vi "Accelerometer Gyroscope and Magnetometer.vi"() -> ()   [LabVIEW 2012, in "Phidget Common.lvlib"]
uses:
  <instrlib>/Phidgets/Phidget Common/Phidget Common.lvlib
  <instrlib>/Phidgets/Phidget Magnetometer/Public/MagnetometerClose.vi
  <instrlib>/Phidgets/Phidget Gyroscope/Public/GyroscopeClose.vi
  <instrlib>/Phidgets/Phidget Accelerometer/Public/AccelerometerClose.vi
  <instrlib>/Phidgets/Phidget Gyroscope/Public/GyroscopeStart.vi
  <instrlib>/Phidgets/Phidget Accelerometer/Public/AccelerometerStart.vi
  <instrlib>/Phidgets/Phidget Magnetometer/Public/MagnetometerStart.vi
  <instrlib>/Phidgets/Phidget Accelerometer/Phidget Accelerometer.lvlib
  <instrlib>/Phidgets/Phidget Gyroscope/Phidget Gyroscope.lvlib
  <instrlib>/Phidgets/Phidget Magnetometer/Phidget Magnetometer.lvlib
panel:
  in  "Device Info":T1={"Serial Number"=-1, "Channel"=0, "Port"=0}
  out "FieldStrength":dbl[](array[numeric])
  out "AngularRate":dbl[](array[numeric])
  out "Acceleration":dbl[](array[numeric])
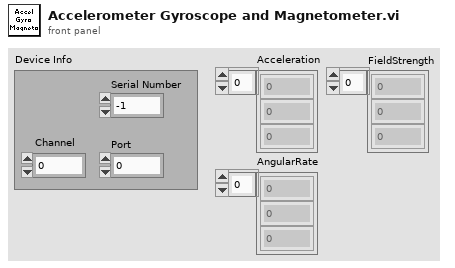
[diagram p1: front panel]
types:
  T1 = cluster{"Serial Number":i32, "Channel":i32, "Port":i32}
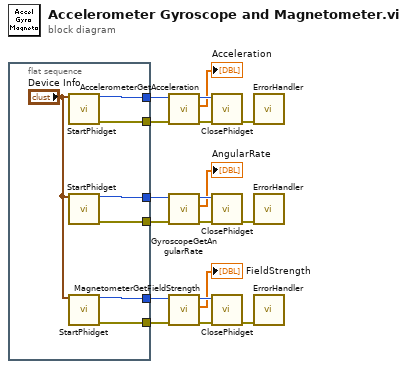
[diagram p0: block diagram]
diagram:
  n1 = flat-sequence {
    tunnel: [w19] -> w18
    tunnel: [w25] -> w17
    tunnel: [w20] -> w16
    tunnel: [w24] -> w15
    tunnel: [w21] -> w14
    tunnel: [w23] -> w13
    frame #0 {
      n2 = call-poly <instrlib>:"StartPhidget.vi"("Device Info"="Device Info") -> ("Phidget ID"=w25:u64, "error out"=w19:errorcluster)  [unwired: 11 in, 2 out]
      n3 = call-poly <instrlib>:"StartPhidget.vi"("Device Info"="Device Info") -> ("Phidget ID"=w24:u64, "error out"=w20:errorcluster)  [unwired: 11 in, 2 out]
      n4 = call-poly <instrlib>:"StartPhidget.vi"("Device Info"="Device Info") -> ("Phidget ID"=w23:u64, "error out"=w21:errorcluster)  [unwired: 11 in, 2 out]
    }
  }
  n5 = call <instrlib>:"AccelerometerGetAcceleration.vi"("error in (no error)"=w18, "Device In"=w17) -> ("error out"=w10:errorcluster, "Acceleration"=→"Acceleration":dbl[], "Device Out"=w9:u64)  [unwired: 6 in]
  n6 = call <instrlib>:"GyroscopeGetAngularRate.vi"("error in (no error)"=w16, "Device In"=w15) -> ("error out"=w12:errorcluster, "AngularRate"=→"AngularRate":dbl[], "Device Out"=w11:u64)  [unwired: 6 in]
  n7 = call <instrlib>:"MagnetometerGetFieldStrength.vi"("error in (no error)"=w14, "Device In"=w13) -> ("error out"=w7:errorcluster, "Magneic Field"=→"FieldStrength":dbl[], "Device Out"=w8:u64)  [unwired: 6 in]
  n8 = call-poly <instrlib>:"ClosePhidget.vi"("error in"=w10, "Device In"=w9) -> ("error out"=w6:errorcluster)  [unwired: 9 in]
  n9 = call-poly <instrlib>:"ClosePhidget.vi"("error in"=w12, "Device In"=w11) -> ("error out"=w4:errorcluster)  [unwired: 9 in]
  n10 = call-poly <instrlib>:"ClosePhidget.vi"("error in"=w7, "Device In"=w8) -> ("error out"=w5:errorcluster)  [unwired: 9 in]
  n11 = call <instrlib>:"ErrorHandler.vi"("error in"=w6) -> ()  [unwired: 9 in, 2 out]
  n12 = call <instrlib>:"ErrorHandler.vi"("error in"=w4) -> ()  [unwired: 9 in, 2 out]
  n13 = call <instrlib>:"ErrorHandler.vi"("error in"=w5) -> ()  [unwired: 9 in, 2 out]
